vi "NewPower_GetCurrent.vi"(3 "error in":errorcluster, 4 "addrPower":T1, 5 "pwr485":refnum<visa-resource-name>="COM3") -> (0 "error out":errorcluster, 2 "Current":dbl)   [LabVIEW 2015]
uses:
  CustomControl/addrPower.ctl
  <vilib>/Instr/_visa.llb/VISA Configure Serial Port (Instr).vi
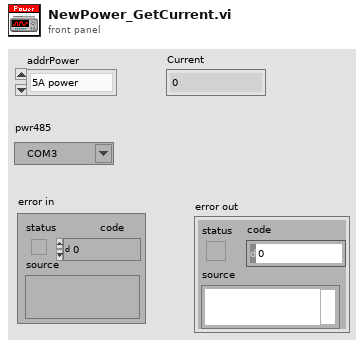
[diagram p1: front panel]
types:
  T1 = typedef "addrPower.ctl" = enum16{"5A power", "300A power"}
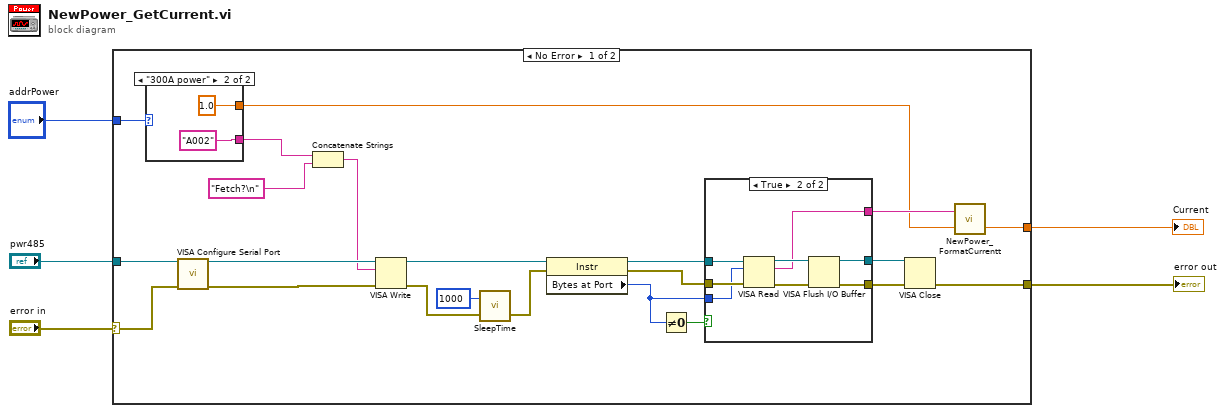
[diagram p0: block diagram]
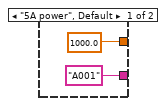
[diagram p3: hidden frame]
diagram:
  n1 = case shown="No Error" "error in" {
    selector: "error in" -> [w7 w42]
    tunnel: "pwr485" -> [w27 _]
    tunnel: "addrPower" -> [w24 _]
    tunnel: [w10 w42] -> w3
    tunnel: [w8 _] -> w2
    frame No Error {
      n2 = case shown="\"300A power\"" w24 {
        tunnel: ["A001" ("format string") "A002" ("format string")] -> w23
        tunnel: [1000.0 ("format string") 1.0 ("format string")] -> w6
        frame "5A power", Default {
        }
        frame "300A power" {
        }
      }
      n3 = call-poly "VISA Configure Serial Port"("VISA resource name"=w27, "error in (no error)"=w7) -> ("VISA resource name out"=w26:refnum<visa-resource-name>, "error out"=w25:errorcluster)  [unwired: 12 in]
      n4 = Concatenate Strings(w23, "Fetch?\n") -> (w21:string)
      n5 = VISA Write(VISA resource name=w26, write buffer=w21, error in (no error)=w25) -> (VISA resource name out=w17:refnum<visa-resource-name>, error out=w20:errorcluster)  [unwired: 1 out]
      n6 = call "SleepTime.vi"("error in (no error)"=w20, "Sleep"=u32 1000) -> ("error out"=w18:errorcluster)  [unwired: 1 in]
      n7 = property class="Instr"(reference=w17, error in=w18) -> (reference out=w15:refnum<visa-resource-name>, error out=w16:errorcluster, "Bytes at Port"=w13:u32)
      n8 = Not Equal To 0?(x=w13) -> (x != 0?=w14:bool)
      n9 = case shown="True" w14 {
        tunnel: w13 -> [_ w35]
        tunnel: w16 -> [w28 w36]
        tunnel: w15 -> [w29 w37]
        tunnel: [_ w32] -> w9
        tunnel: [w29 w31] -> w12
        tunnel: [w28 w30] -> w11
        frame False {
        }
        frame True {
          n10 = VISA Read(VISA resource name=w37, byte count=w35, error in (no error)=w36) -> (VISA resource name out=w34:refnum<visa-resource-name>, read buffer=w32:string, error out=w33:errorcluster)  [unwired: 1 out]
          n11 = VISA Flush I/O Buffer(VISA resource name=w34, error in (no error)=w33) -> (VISA resource name out=w31:refnum<visa-resource-name>, error out=w30:errorcluster)  [unwired: 1 in]
        }
      }
      n12 = VISA Close(VISA resource name=w12, error in (no error)=w11) -> (error out=w10:errorcluster)
      n13 = call "NewPower_FormatCurrentt.vi"("y"=w6, "FetchStr"=w9) -> ("Current"=w8:dbl)  [unwired: 1 in]
    }
    frame Error {
    }
  }
  "error out" <- w3
  "Current" <- w2
